vi "tesst_pos_control.vi"() -> ()   [LabVIEW 2020]
panel:
  out "On target":bool
  out "output variable":dbl
  in  "Error":dbl
  in  "mindemand":dbl
  in  "threshold":dbl
  in  "maxdemand":dbl
  in  "deadband":dbl
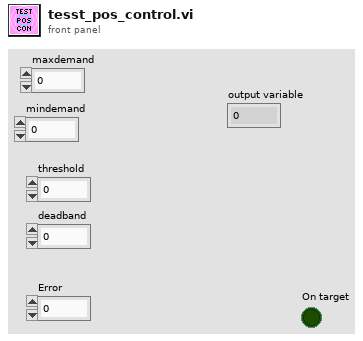
[diagram p1: front panel]
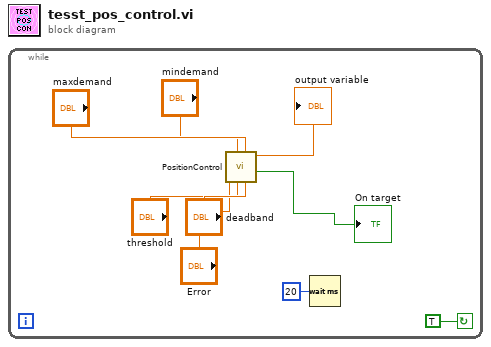
[diagram p0: block diagram]
diagram:
  n1 = while {
    stop <- TRUE continue-if-true
    n2 = call "PositionControl.vi"("deadband"="deadband", "maxdemand"="maxdemand", "threshold"="threshold", "mindemand"="mindemand", "Error"="Error") -> ("on target"=→"On target":bool, "output variable"=→"output variable":dbl)  [unwired: 5 in]
    n3 = Wait (ms)(milliseconds to wait=u32 20) -> ()  [unwired: 1 out]
  }
